vi "read_voltage.vi"(1 "Channel":i32 min=0 max=15) -> (0 "Voltage":dbl)   [LabVIEW 2011]
uses:
  globals.vi
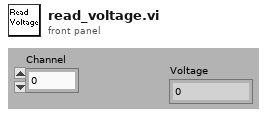
[diagram p1: front panel]
types:
  T1 = cluster{"Relay Card Slots":cluster{"Card 1":u16, "Card 2":u16, "Card 3":u16, "Card 4":u16, "Card 5":u16}, "A/D Card Slots":cluster{"Scanner":u16, "High-Speed A/D":u16, "Timer":u16}, "D/A Cards":cluster{"Quad (10-bit) D/A Card Slots":cluster{"Card 1":u16, "Card 2":u16, "Card 3":u16, "Card 4":u16, "Card 5":u16}, "Single (12-bit) D/A Card Slot":cluster{"Card 6":u16}}}
  T2 = cluster{"Scanner":u16, "High-Speed A/D":u16, "Timer":u16}
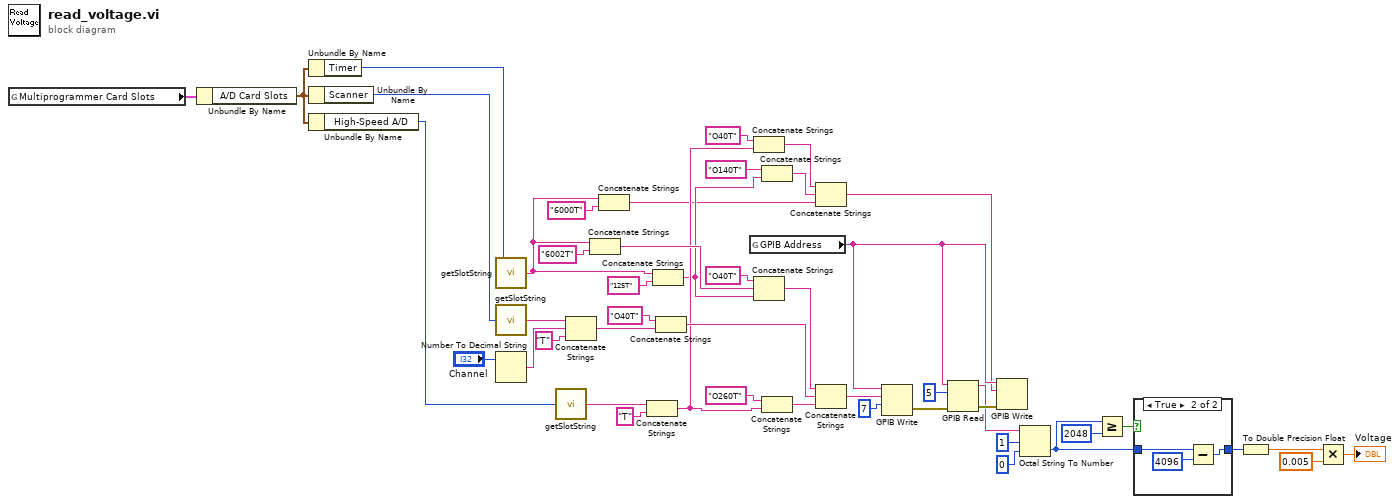
[diagram p0: block diagram]
diagram:
  n1 = global read "globals.vi" "Multiprogrammer Card Slots"() -> (w5:T1)
  n2 = Unbundle By Name(w5) -> ("A/D Card Slots"=w2:T2)
  n3 = Unbundle By Name(w2) -> ("Timer"=w4:u16)
  n4 = Unbundle By Name(w2) -> ("Scanner"=w3:u16)
  n5 = Unbundle By Name(w2) -> ("High-Speed A/D"=w1:u16)
  n6 = call "getSlotString.vi"("Slot"=w4) -> ("string"=w11:string)
  n7 = call "getSlotString.vi"("Slot"=w3) -> ("string"=w26:string)
  n8 = Number To Decimal String(number="Channel") -> (decimal integer string=w25:string)  [unwired: 1 out]
  n9 = call "getSlotString.vi"("Slot"=w1) -> ("string"=w21:string)
  n10 = Concatenate Strings(w26, w25, "T" ("string")) -> (w24:string)
  n11 = Concatenate Strings(w11, "6002T" ("data")) -> (w29:string)
  n12 = Concatenate Strings(w11, "6000T" ("data")) -> (w7:string)
  n13 = Concatenate Strings(w21, "T" ("string")) -> (w15:string)
  n14 = Concatenate Strings(w11, "125T" ("data")) -> (w12:string)
  n15 = Concatenate Strings("O40T" ("data"), w24) -> (w18:string)
  n16 = global read "globals.vi" "GPIB Address"() -> (w33:string)
  n17 = Concatenate Strings("O40T" ("data"), w15) -> (w9:string)
  n18 = Concatenate Strings("O40T" ("data"), w29, w12) -> (w19:string)
  n19 = Concatenate Strings("O140T" ("data"), w12) -> (w8:string)
  n20 = Concatenate Strings("O260T" ("string"), w15) -> (w17:string)
  n21 = Concatenate Strings(w9, w8, w7) -> (w6:string)
  n22 = Concatenate Strings(w19, w18, w17) -> (w36:string)
  n23 = GPIB Write(0:w33, 1:w36, 2:i16 7 ("mode (0)")) -> (6:w47:errorcluster)  [unwired: 1 in, 2 out]
  n24 = GPIB Read(0:w33, 1:5 ("byte count"), 3:w47) -> (5:w44:string, 7:w46:errorcluster)  [unwired: 3 out]
  n25 = GPIB Write(0:w33, 1:w6, 3:w46) -> ()  [unwired: 4 out]
  n26 = Octal String To Number(2:0 ("default (0 U32)"), 3:1 ("offset"), 4:w44) -> (0:w38:i32)  [unwired: 1 out]
  n27 = Greater Or Equal?(x=w38, y=2048) -> (x >= y?=w39:bool)
  n28 = case shown="True" w39 {
    tunnel: w38 -> [w48 w49]
    tunnel: [w48 w51] -> w37
    frame False {
    }
    frame True {
      n29 = Subtract(x=w49, y=4096 ("x")) -> (x-y=w51:i32)
    }
  }
  n30 = To Double Precision Float(number=w37) -> (double precision float=w43:dbl)
  n31 = Multiply(x=w43, y=0.005) -> (x*y=→"Voltage":dbl)
